vi "Turn.vi"(10 "Current Heading":dbl format="%.2f", 11 "Desired Heading":dbl) -> (3 "Motor Vals":dbl format="%.2f")   [LabVIEW 2016]
uses:
  <vilib>/addons/control/pid/pid.llb/PID Advanced (DBL).vi
  <vilib>/addons/control/pid/NI_PID_pid.lvlib
panel:
  in  "PID gains":T1={"proportional gain (Kc)"=0.8, "integral time (Ti, min)"=0.01, "derivative time (Td, min)"=0.0} {"derivative time (Td, min)" format="%.3f"; "integral time (Ti, min)" format="%.3f"; "proportional gain (Kc)" format="%.3f"}
  in  "gamma":dbl format="%.2f"
  in  "alpha":dbl=nan format="%.2f"
  in  "beta":dbl=1.0 format="%.2f"
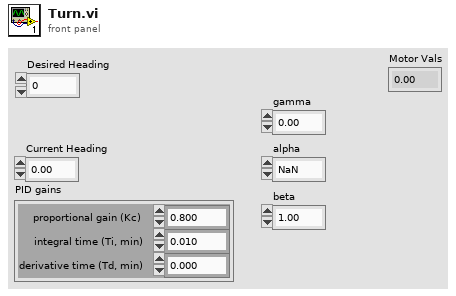
[diagram p1: front panel]
types:
  T1 = cluster{"proportional gain (Kc)":dbl, "integral time (Ti, min)":dbl, "derivative time (Td, min)":dbl}
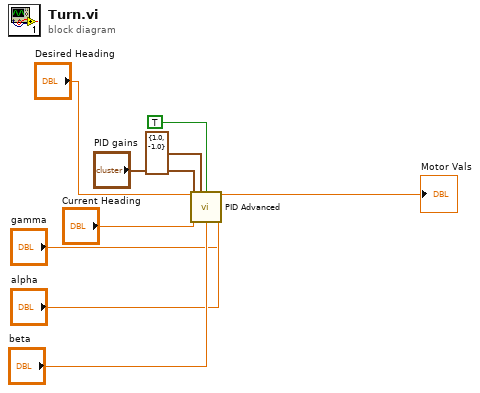
[diagram p0: block diagram]
diagram:
  n1 = call-poly <vilib>:"PID Advanced.vi"("setpoint"="Desired Heading", "output range"=cluster{"output high":dbl, "output low":dbl} {"output high"=1.0, "output low"=-1.0}, "auto? (T)"=TRUE, "process variable"="Current Heading", "gamma"="gamma", "alpha"="alpha", "PID gains"="PID gains", "beta"="beta") -> ("output"=→"Motor Vals":dbl)  [unwired: 6 in, 1 out]
